vi "Main_Sweep_Demo Setting.vi"() -> ()   [LabVIEW 2016]
uses:
  Hardware/Ctl_SetParameter(Value).ctl
  <instrlib>/Zurich Instruments LabOne/Public/Configure/ziSetValueDoubleArray.vi
  Hardware/General.lvlib
  <instrlib>/Zurich Instruments LabOne/Zurich Instruments LabOne.lvlib
panel:
  out "Done?":bool
  out "HDAWG Connection for this demo":string="Object:\n[Trig of Channel group 1] of HDAWG receives external trigger to start generation.\n[Mark  of Channel group 1] of HDAWG generates \"Sample Trigger\" for UHFLI, in order to save bandwidth and achieve high Transfer Rate(7.031M Sa/s).\n\nConnection:\n[Trig of Channel group 1] of HDAWG to [Trigger 3] of UHF.\n[Wave of Channel group 1] of HDAWG to [Signal Input 1] of UHF."
  out "HDAWG Device":string
  out "UHF Connection for this demo":string="Object:\n[Ref/Trigger 2] of UHF will be used as external trigger source(e.g. Delayer).\n\nConnection:\n[Ref/Trigger 2] of UHF connects to [Trig of Channel group 1] of HDAWG."
  out "UHF Device":string
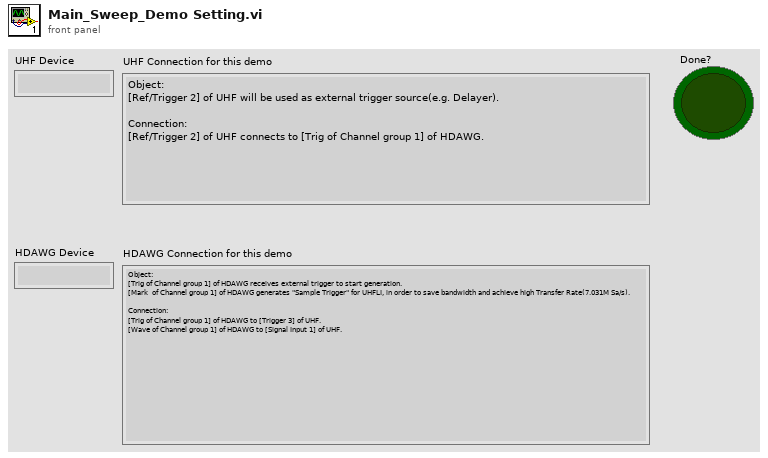
[diagram p1: front panel]
types:
  T1 = typedef "General.lvlib/Ctl_SetParameter(Value).ctl" = cluster{"Path":string, "Value":dbl, "comment":string}
  T2 = typedef "Hardware_DeviceAddresses.ctl" = cluster{"ZI Device Name":string[][], "MW Source":T3, "Trigger Delayer VISA":refnum<visa-resource-name>}
  T3 = typedef "Microwave Source.lvlib/MW_ctl_DeviceHandles..ctl" = cluster{"LO VISA":refnum<visa-resource-name>, "Probe VISA":refnum<visa-resource-name>, "Qubits":refnum<visa-resource-name>[]}
  T4 = typedef "Zurich Instruments LabOne.lvlib/ziTypeHandle.ctl" = cluster{"handleValid":bool, "Conn":u64, "Path Prefix":string, "Handle":u64, "Connected":bool, "Clockbase(s)":dbl}
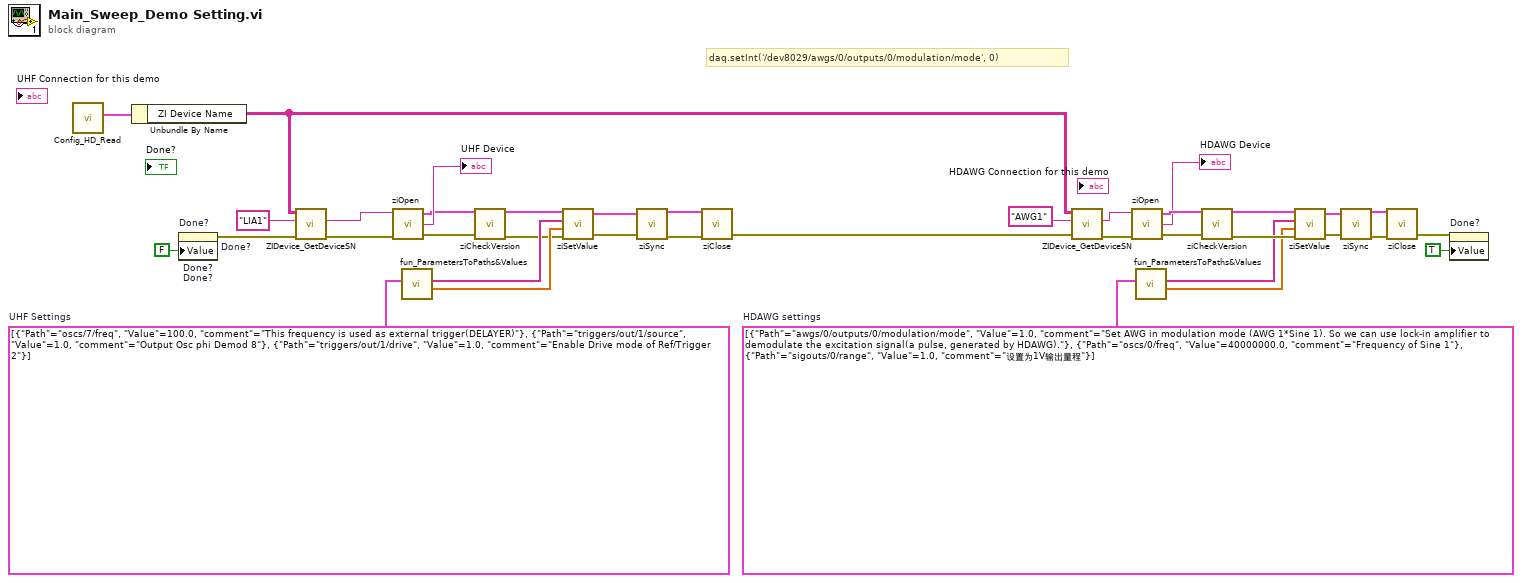
[diagram p0: block diagram]
diagram:
  w10 = T1[] [{"Path"="awgs/0/outputs/0/modulation/mode", "Value"=1.0, "comment"="Set AWG in modulation mode (AWG 1*Sine 1). So we can use lock-in amplifier to demodulate the excitation signal(a pulse, generated by HDAWG)."}, {"Path"="oscs/0/freq", "Value"=40000000.0, "comment"="Frequency of Sine 1"}, {"Path"="sigouts/0/range", "Value"=1.0, "comment"="设置为1V输出量程"}]  # HDAWG settings
  w29 = T1[] [{"Path"="oscs/7/freq", "Value"=100.0, "comment"="This frequency is used as external trigger(DELAYER)"}, {"Path"="triggers/out/1/source", "Value"=1.0, "comment"="Output Osc phi Demod 8"}, {"Path"="triggers/out/1/drive", "Value"=1.0, "comment"="Enable Drive mode of Ref/Trigger 2"}]  # UHF Settings
  # "daq.setInt('/dev8029/awgs/0/outputs/0/modulation/mode', 0)"
  n1 = call "Config_HD_Read.vi"() -> ("Dev Address"=w40:T2)  [unwired: 11 in]
  n2 = Unbundle By Name(w40) -> ("ZI Device Name"=w12:string[][])
  n3 = property on="Done?" class="Bool (strict)"("Value"=FALSE ("Done?")) -> ()  [unwired: 2 in, 2 out]
  n4 = property on="Done?" class="Bool (strict)"("Value"=FALSE ("Done?")) -> ()  [unwired: 2 in, 2 out]
  n5 = property on="Done?" class="Bool (strict)"("Value"=FALSE ("Done?")) -> ()  [unwired: 2 in, 2 out]
  n6 = property on="Done?" class="Bool (strict)"("Value"=FALSE ("Done?")) -> (error out=w7:errorcluster)  [unwired: 2 in, 1 out]
  n7 = call "ZIDevice_GetDeviceSN.vi"("error in (no error)"=w7, "alias"="LIA1", "Hardware Handle.Device Name"=w12) -> ("error out"=w31:errorcluster, "Device SN"=w30:string)  [unwired: 7 in]
  n8 = call <instrlib>:"ziOpen.vi"("Error In"=w31, "Address"=w30) -> ("Error Out"=w35:errorcluster, "Selected Device"=→"UHF Device":string, "HandleOut"=w32:T4)  [unwired: 2 out]
  n9 = call "fun_ParametersToPaths&Values.vi"("Parameters"=w29) -> ("Values"=w38:dbl[], "Paths"=w37:string[])  [unwired: 9 in]
  n10 = call <instrlib>:"ziCheckVersion.vi"("Handle In"=w32, "Error In"=w35) -> ("Handle Out"=w33:T4, "Error Out"=w34:errorcluster)  [unwired: 11 in, 1 out]
  n11 = call-poly <instrlib>:"ziSetValue.vi"("Error In"=w34, "Values"=w38, "Paths"=w37, "Handle In"=w33) -> ("Error Out"=w25:errorcluster, "Handle Out"=w28:T4)  [unwired: 1 in]
  n12 = call <instrlib>:"ziSync.vi"("Handle In"=w28, "Error In"=w25) -> ("Handle Out"=w27:T4, "Error Out"=w26:errorcluster)  [unwired: 12 in]
  n13 = call <instrlib>:"ziClose.vi"("Error In"=w26, "Handle In"=w27) -> ("Error Out"=w11:errorcluster)  [unwired: 2 in, 1 out]
  n14 = call "ZIDevice_GetDeviceSN.vi"("error in (no error)"=w11, "alias"="AWG1", "Hardware Handle.Device Name"=w12) -> ("error out"=w19:errorcluster, "Device SN"=w20:string)  [unwired: 7 in]
  n15 = call <instrlib>:"ziOpen.vi"("Error In"=w19, "Address"=w20) -> ("Error Out"=w15:errorcluster, "Selected Device"=→"HDAWG Device":string, "HandleOut"=w18:T4)  [unwired: 2 out]
  n16 = call "fun_ParametersToPaths&Values.vi"("Parameters"=w10) -> ("Values"=w9:dbl[], "Paths"=w8:string[])  [unwired: 9 in]
  n17 = call <instrlib>:"ziCheckVersion.vi"("Handle In"=w18, "Error In"=w15) -> ("Handle Out"=w17:T4, "Error Out"=w16:errorcluster)  [unwired: 11 in, 1 out]
  n18 = call-poly <instrlib>:"ziSetValue.vi"("Error In"=w16, "Values"=w9, "Paths"=w8, "Handle In"=w17) -> ("Error Out"=w24:errorcluster, "Handle Out"=w21:T4)  [unwired: 1 in]
  n19 = call <instrlib>:"ziSync.vi"("Handle In"=w21, "Error In"=w24) -> ("Handle Out"=w22:T4, "Error Out"=w23:errorcluster)  [unwired: 12 in]
  n20 = call <instrlib>:"ziClose.vi"("Error In"=w23, "Handle In"=w22) -> ("Error Out"=w1:errorcluster)  [unwired: 2 in, 1 out]
  n21 = property on="Done?" class="Bool (strict)"(error in=w1, "Value"=TRUE ("Done?")) -> ()  [unwired: 1 in, 2 out]
